vi "FTW-SQLite-LibraryFilepath.vi"(8 "error in":errorcluster, 10 "Rediscover library?":bool) -> (0 "error out":errorcluster, 1 "SQLite Version":string, 2 "SQLite Library Filepath":path)   [LabVIEW 2013, in "FTW-SQLite-Connector.lvclass"]
uses:
  FTW-SQLite-Connector.lvclass
  error/FTW-ERR-ThrowError.vi
  error/FTW-ERR-NoErrorConstant.vi
  error/FTW-ERR-CallChain.vi
  string/FTW-STR-ReplaceWhitespace.vi
  lib/FTWLib-SQLite3-Win32.dll
  lib/FTWLib-SQLite3-Win64.dll
  lib/FTWLib-SQLite3-LinuxRT.so
panel:
  # "Inputs"
  # "Outputs"
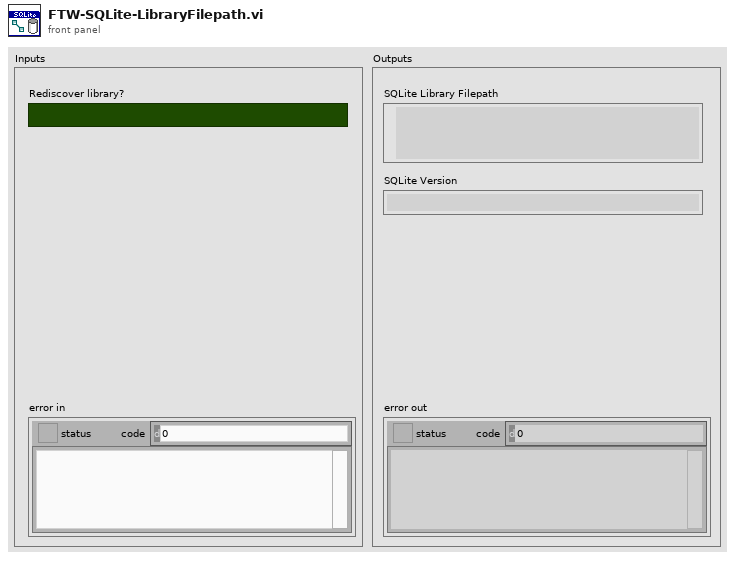
[diagram p1: front panel]
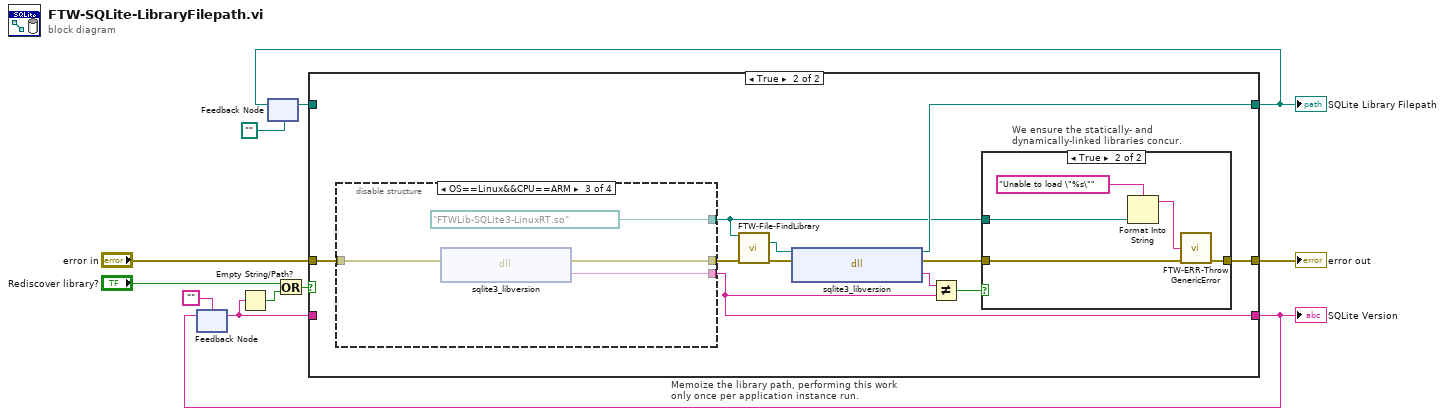
[diagram p0: block diagram]
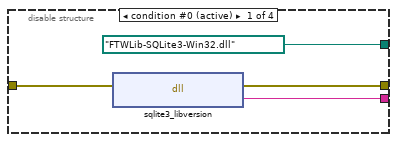
[diagram p4: hidden frame]
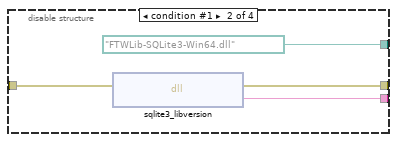
[diagram p5: hidden frame]
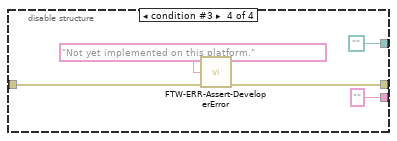
[diagram p6: hidden frame]
diagram:
  n1 = feedback #1("") -> (w4:string)
  n2 = Empty String/Path?(string/path=w4) -> (empty?=w3:bool)
  n3 = feedback #2(path "") -> (w9:path)
  n4 = Or(x="Rediscover library?", y=w3) -> (x .or. y?=w5:bool)
  n5 = case "Memoize the library path, performing this work only once per application instance run." shown="True" w5 {
    tunnel: [w14 w24] -> w8
    tunnel: "error in" -> [w13 w25]
    tunnel: [w12 w19] -> w7
    tunnel: [w13 w16] -> w10
    tunnel: w9 -> [w14 _]
    tunnel: w4 -> [w12 _]
    frame False {
    }
    frame True {
      n6 = disable-structure shown="OS==Linux&&CPU==ARM" {
        disable-tunnel: [path "FTWLib-SQLite3-Win32.dll" path "FTWLib-SQLite3-Win64.dll" path "FTWLib-SQLite3-LinuxRT.so" path ""] -> w15
        disable-tunnel: [w33 w37 w41 w47] -> w23
        disable-tunnel: w25 -> [w34 w38 w42 w48]
        disable-tunnel: [w32 w36 w40 "" ("Return Value")] -> w19
        frame condition #0 (active) {
          n7 = dll-call lib="C:/Users/Jack/repo/ftw-master/ftw/src/core/database/lib/FTWLib-SQLite3-Win32.dll" fn="sqlite3_libversion" label="FTWLib-SQLite3-Win32.dll"(error in=w34) -> (error out=w33:errorcluster, "Return Value"=w32:string)  [unwired: 2 in, 1 out]
        }
        frame condition #1 {
          n8 = dll-call lib="C:/Users/Jack/repo/ftw-master/ftw/src/core/database/lib/FTWLib-SQLite3-Win64.dll" fn="sqlite3_libversion" label="FTWLib-SQLite3-Win64.dll"(error in=w38) -> (error out=w37:errorcluster, "Return Value"=w36:string)  [unwired: 2 in, 1 out]
        }
        frame condition #2 {
          n9 = dll-call lib="C:/Users/Jack/repo/ftw-master/ftw/src/core/database/lib/FTWLib-SQLite3-LinuxRT.so" fn="sqlite3_libversion" label="FTWLib-SQLite3-LinuxRT.so"(error in=w42) -> (error out=w41:errorcluster, "Return Value"=w40:string)  [unwired: 2 in, 1 out]
        }
        frame condition #3 {
          n10 = call "FTW-ERR-Assert-DeveloperError.vi"("Reason this error should never happen"="Not yet implemented on this platform.", "error in"=w48) -> ("error out"=w47:errorcluster)  [unwired: 13 in]
        }
      }
      n11 = call "FTW-File-FindLibrary.vi"("Library File Pattern"=w15, "error in"=w23) -> ("Library Filepath"=w21:path, "error out"=w22:errorcluster)  [unwired: 12 in]
      n12 = dll-call lib="?" fn="sqlite3_libversion"(path in=w21, error in=w22) -> (path out=w24:path, error out=w17:errorcluster, "Return Value"=w20:string)  [unwired: 1 in]
      n13 = Not Equal?(x=w20, y=w19) -> (x != y?=w18:bool)
      n14 = case "We ensure the statically- and\ndynamically-linked libraries concur." shown="True" w18 {
        tunnel: w17 -> [w26 w31]
        tunnel: [w26 w30] -> w16
        tunnel: w15 -> [_ w29]
        frame False {
        }
        frame True {
          n15 = Format Into String(format string="Unable to load \"%s\"", w29) -> (resulting string=w28:string)  [unwired: 2 in, 1 out]
          n16 = call "FTW-ERR-ThrowGenericError.vi"("Error Message"=w28, "error in"=w31) -> ("error out"=w30:errorcluster)  [unwired: 13 in]
        }
      }
    }
  }
  "error out" <- w10
  "SQLite Library Filepath" <- w8
  "SQLite Version" <- w7
  n17 = feedback-in #1(w7) -> ()
  n18 = feedback-in #2(w8) -> ()
